vi "Lissage de signal_base.vi"() -> ()   [LabVIEW 2018]
panel:
  in  "stop":bool
  out "Graphe déroulant":cluster{dbl, dbl}(graph)
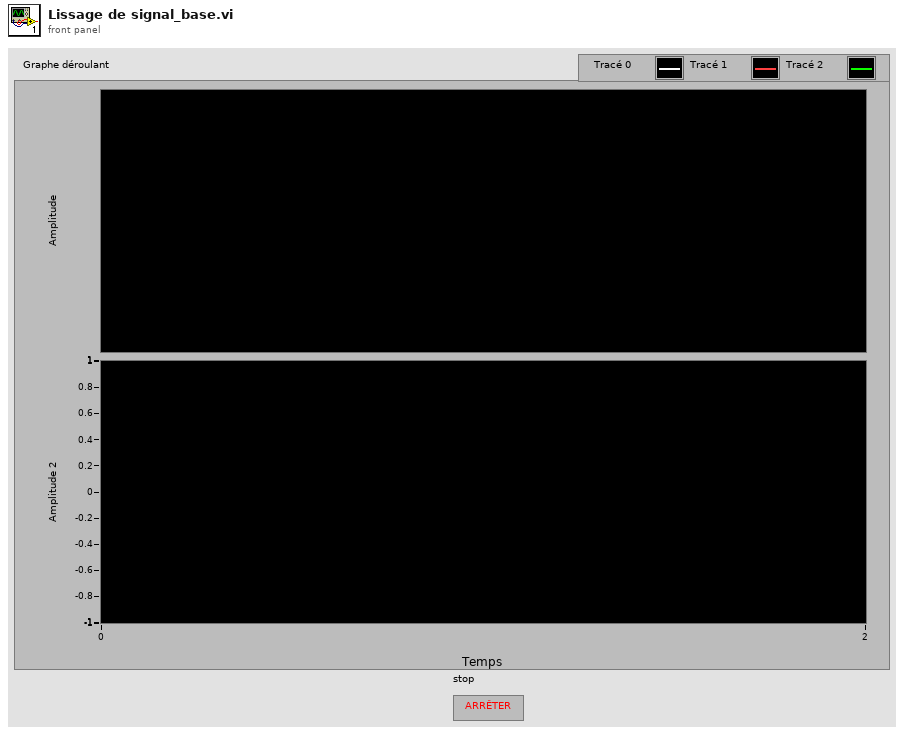
[diagram p1: front panel]
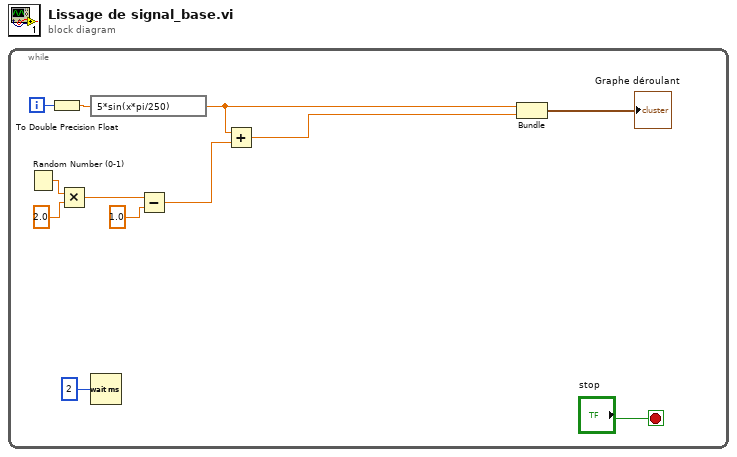
[diagram p0: block diagram]
diagram:
  n1 = while {
    i -> [w9]
    stop <- "stop" stop-if-true
    n2 = Random Number (0-1)() -> (number: 0 to 1=w7:dbl)
    n3 = To Double Precision Float(number=w9) -> (double precision float=w11:dbl)
    n4 = Multiply(x=w7, y=2.0) -> (x*y=w5:dbl)
    n5 = expression code="5*sin(x*pi/250)"(w11) -> (w2:dbl)
    n6 = Wait (ms)(milliseconds to wait=u32 2 ("attente (ms)")) -> ()  [unwired: 1 out]
    n7 = Subtract(x=w5, y=1.0) -> (x-y=w3:dbl)
    n8 = Add(x=w2, y=w3) -> (x+y=w1:dbl)
    n9 = Bundle(w2, w1) -> (→"Graphe déroulant":cluster{dbl, dbl})  [unwired: 1 in]
  }
